vi "Calculate Steps.vi"(4 "Blueprints":T4 {"Robot Building Costs"."Geode"."Mineral" items=["Ore", "Clay", "Obsidian", "Geode", "Open Geode"]; "Robot Building Costs"."Obsidian"."Mineral" items=["Ore", "Clay", "Obsidian", "Geode", "Open Geode"]; "Robot Building Costs"."Clay"."Mineral" items=["Ore", "Clay", "Obsidian", "Geode", "Open Geode"]; "Robot Building Costs"."Ore"."Mineral" items=["Ore", "Clay", "Obsidian", "Geode", "Open Geode"]}, 5 "#Total Time":u32, 9 "Initial Status":T1) -> (3 "Steps":map{string, T1}(c390))   [LabVIEW 2020, in "AoC 2022.lvlib"]
uses:
  AoC 2022.lvlib
  Step.ctl
  Inventory.ctl
  Robot Factory.ctl
  Blueprints.ctl
  Robot Building Costs.ctl
  Cost.ctl
  Mineral.ctl
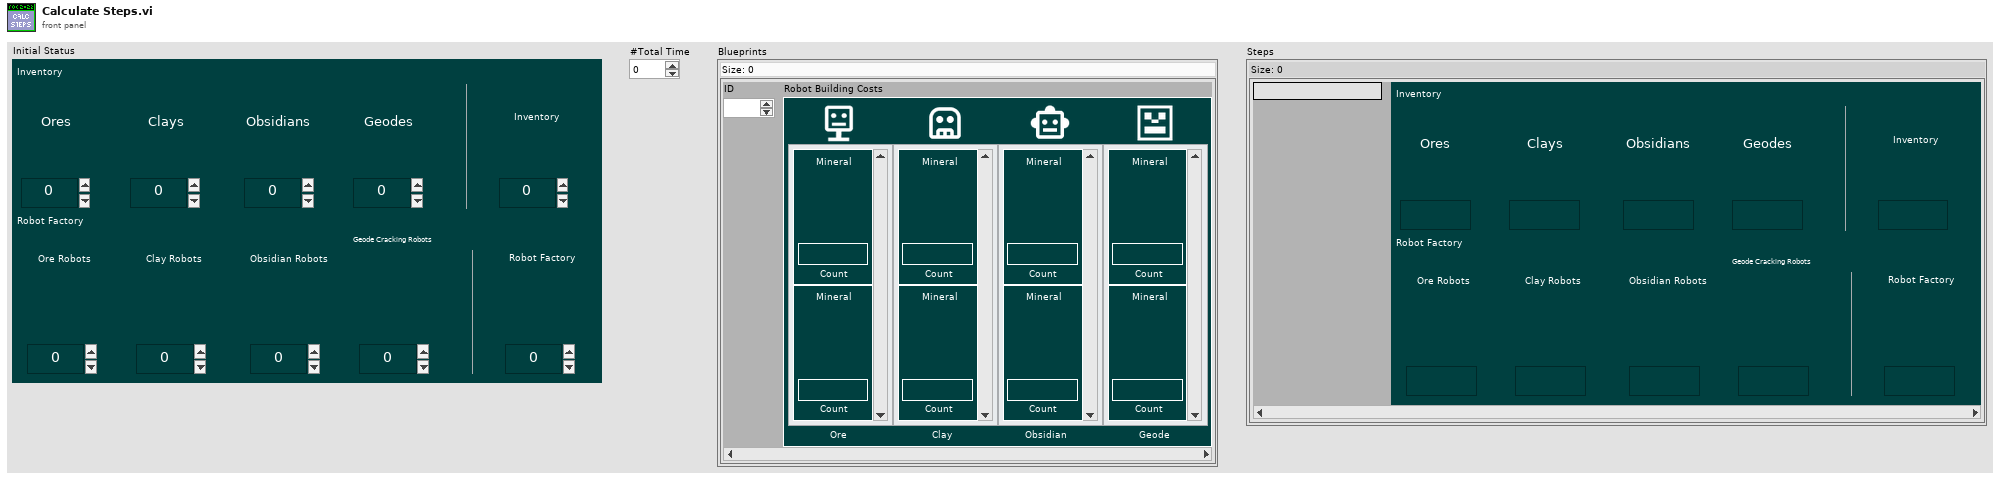
[diagram p1: front panel]
types:
  T1 = typedef "AoC 2022.lvlib/Step.ctl" = cluster{"Inventory":T2, "Robot Factory":T3}
  T2 = typedef "AoC 2022.lvlib/Inventory.ctl" = cluster{"Ores":u32, "Clays":u32, "Obsidians":u32, "Geodes":u32, "Inventory":u32}
  T3 = typedef "AoC 2022.lvlib/Robot Factory.ctl" = cluster{"Ore Robots":u32, "Clay Robots":u32, "Obsidian Robots":u32, "Geode Cracking Robots":u32, "Robot Factory":u32}
  T4 = typedef "AoC 2022.lvlib/Blueprints.ctl" = map{i32, T5}
  T5 = typedef "AoC 2022.lvlib/Robot Building Costs.ctl" = cluster{"Ore":T6[], "Clay":T6[], "Obsidian":T6[], "Geode":T6[]}
  T6 = typedef "AoC 2022.lvlib/Cost.ctl" = cluster{"Mineral":T7, "Count":u32}
  T7 = typedef "AoC 2022.lvlib/Mineral.ctl" = u16
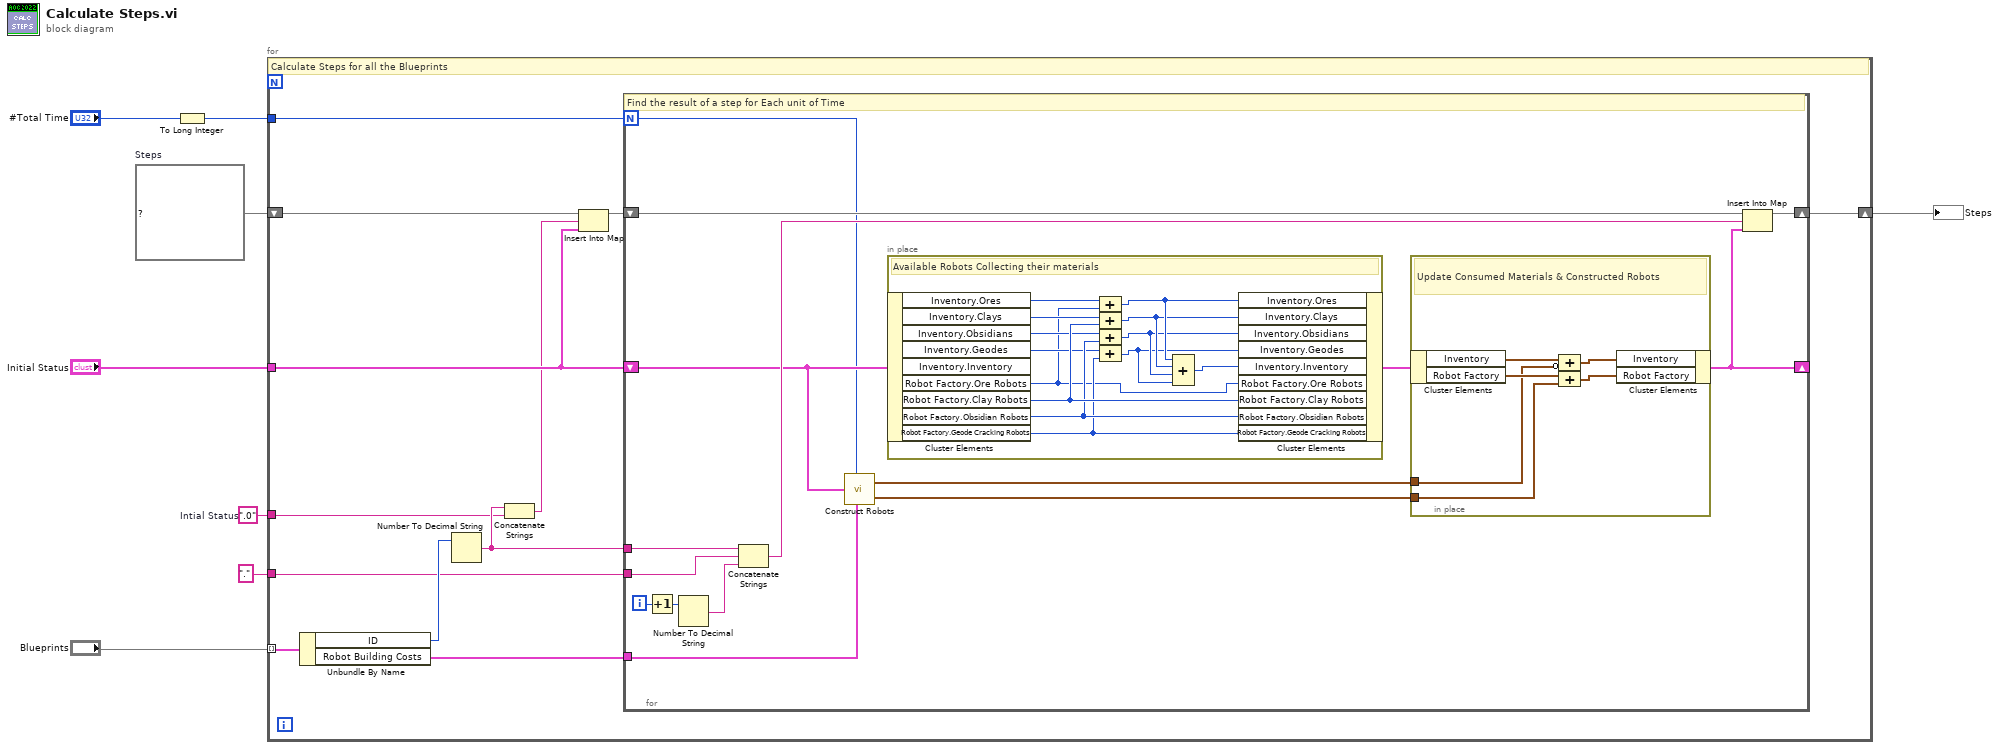
[diagram p0: block diagram]
diagram:
  w3 = ".0"  # Intial Status
  w5 = map{string, T1} {}  # Steps
  n1 = To Long Integer(number="#Total Time") -> (32bit integer=w6:i32)
  n2 = for {
    tunnel: "Blueprints" -> [w18] mode=indexing
    tunnel: w6 -> [w20]
    shift-right: [w19] -> w4
    shift-left: w5 -> [w16]
    tunnel: w3 -> [w11]
    tunnel: "Initial Status" -> [w14]
    tunnel: "." -> [w9]
    # "Calculate Steps for all the Blueprints"
    n3 = Unbundle By Name(w18) -> ("ID"=w13:i32, "Robot Building Costs"=w17:T5)
    n4 = Number To Decimal String(number=w13) -> (decimal integer string=w12:string)  [unwired: 1 in]
    n5 = Concatenate Strings(w12, w11) -> (w10:string)
    n6 = Insert Into Map(map in=w16, key=w10, value=w14) -> (map out=w15:map{string, T1})  [unwired: 2 out]
    n7 = for {
      N: w20 -> [w26]
      shift-right: [w35] -> w19
      shift-left: w15 -> [w34]
      tunnel: w17 -> [w28]
      shift-right: [w24] -> _
      shift-left: w14 -> [w27]
      tunnel: w12 -> [w31]
      tunnel: w9 -> [w29]
      i -> [w33]
      # "Find the result of a step for Each unit of Time"
      n8 = Increment(x=w33) -> (x+1=w21:i32)
      n9 = Number To Decimal String(number=w21) -> (decimal integer string=w32:string)  [unwired: 1 in]
      n10 = Concatenate Strings(w31, w29, w32) -> (w30:string)
      n11 = call "Construct Robots.vi"("Total Steps to be Executed"=w26, "Factory Status"=w27, "Robot Building Costs"=w28) -> ("Consumed Materials"=w23:T2, "Constructed Robots"=w22:T3)  [unwired: 2 in]
      n12 = in-place {
        # "Available Robots Collecting their materials"
        n13 = in-place-cluster #1(w27) -> ("Inventory.Ores"=w54:u32, "Inventory.Clays"=w53:u32, "Inventory.Obsidians"=w51:u32, "Inventory.Geodes"=w49:u32, "Robot Factory.Ore Robots"=w42:u32, "Robot Factory.Clay Robots"=w52:u32, "Robot Factory.Obsidian Robots"=w50:u32, "Robot Factory.Geode Cracking Robots"=w48:u32)  [unwired: 1 out]
        n14 = Compound Arithmetic op=ADD(w54, w42) -> (w47:u32)
        n15 = Compound Arithmetic op=ADD(w53, w52) -> (w46:u32)
        n16 = Compound Arithmetic op=ADD(w51, w50) -> (w45:u32)
        n17 = Compound Arithmetic op=ADD(w49, w48) -> (w44:u32)
        n18 = Compound Arithmetic op=ADD(w47, w46, w45, w44) -> (w43:u32)
        n19 = in-place-cluster #1("Inventory.Ores"=w47, "Inventory.Clays"=w46, "Inventory.Obsidians"=w45, "Inventory.Geodes"=w44, "Inventory.Inventory"=w43, "Robot Factory.Ore Robots"=w42, "Robot Factory.Clay Robots"=w52, "Robot Factory.Obsidian Robots"=w50, "Robot Factory.Geode Cracking Robots"=w48) -> (w25:T1)
      }
      n20 = in-place {
        in-place-border: w23 -> [w37]
        in-place-border: w22 -> [w36]
        # "Update Consumed Materials & Constructed Robots"
        n21 = in-place-cluster #2(w25) -> ("Inventory"=w41:T2, "Robot Factory"=w40:T3)
        n22 = Compound Arithmetic op=ADD(w41, invert w37) -> (w39:T2)
        n23 = Compound Arithmetic op=ADD(w40, w36) -> (w38:T3)
        n24 = in-place-cluster #2("Inventory"=w39, "Robot Factory"=w38) -> (w24:T1)
      }
      n25 = Insert Into Map(map in=w34, key=w30, value=w24) -> (map out=w35:map{string, T1})  [unwired: 2 out]
    }
  }
  "Steps" <- w4
